vi "calcNoSteps.vi"(1 "inc (um)":dbl, 2 "init pos (mm)":dbl, 3 "fin pos (mm)":dbl) -> (0 "no. steps":i16)   [LabVIEW 2015]
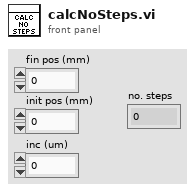
[diagram p1: front panel]
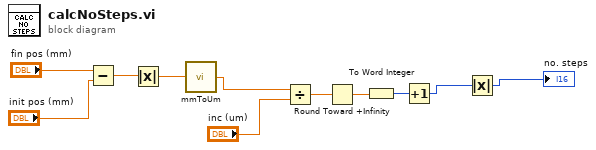
[diagram p0: block diagram]
diagram:
  n1 = Subtract(x="fin pos (mm)", y="init pos (mm)") -> (x-y=w9:dbl)
  n2 = Absolute Value(x=w9) -> (abs(x)=w8:dbl)
  n3 = call "mmToUm.vi"("distance (mm)"=w8) -> ("distance (um)"=w7:dbl)
  n4 = Divide(x=w7, y="inc (um)") -> (x/y=w5:dbl)
  n5 = Round Toward +Infinity(x=w5) -> (ceil(x): smallest int >= x=w4:dbl)
  n6 = To Word Integer(number=w4) -> (16bit integer=w3:i16)
  n7 = Increment(x=w3) -> (x+1=w2:i16)
  n8 = Absolute Value(x=w2) -> (abs(x)=→"no. steps":i16)
